vi "CRYGet Phase Index.vi"(10 "SelectedRow":i32[](array[numeric]), 11 "Legend Ref":refnum<vi>) -> (2 "CurveLibIndex":i32[](array[numeric]), 3 "LegendIndex":i32[](array[numeric]))   [LabVIEW 2013]
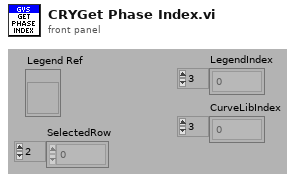
[diagram p1: front panel]
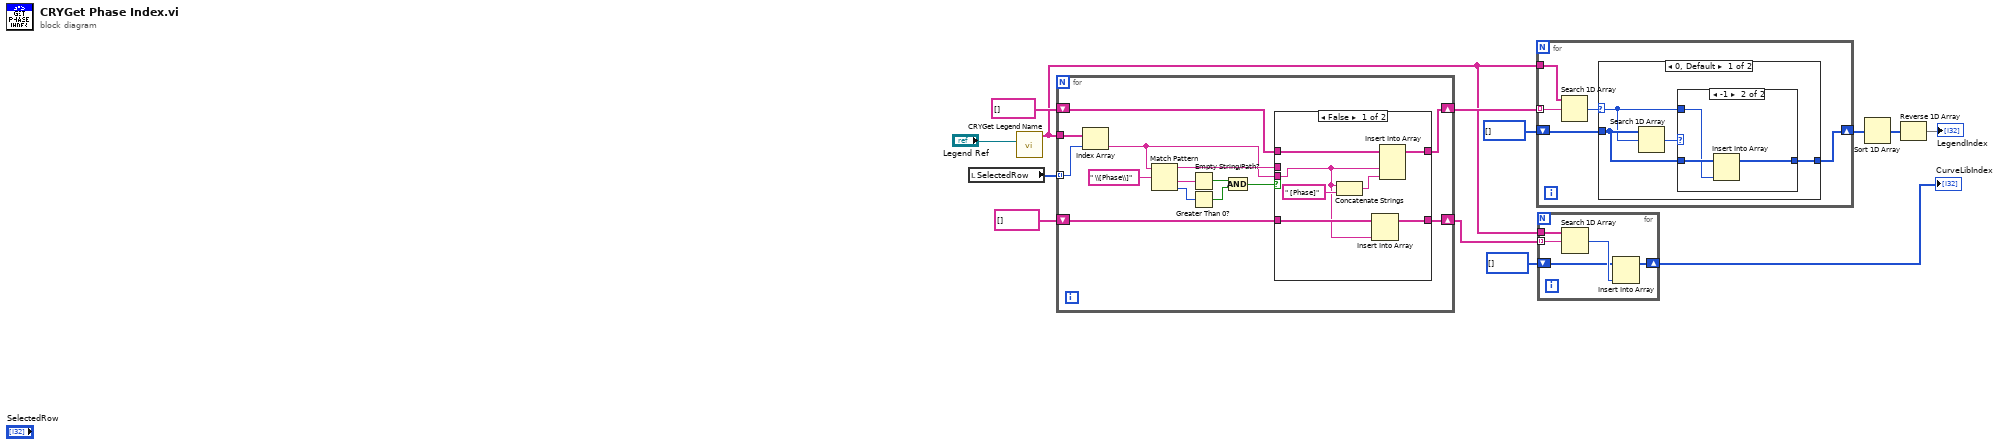
[diagram p0: block diagram]
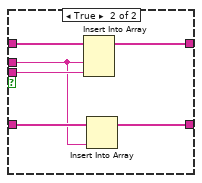
[diagram p4: hidden frame]
diagram:
  n1 = local read "SelectedRow"() -> (w13:i32[])
  n2 = call "CRYGet Legend Name.vi"("MCListbox Refnum"="Legend Ref") -> ("Names Out"=w3:string[])  [unwired: 10 in]
  n3 = for {
    tunnel: w13 -> [w26] mode=indexing
    tunnel: w3 -> [w27]
    shift-right: [w16] -> w11
    shift-left: string[] [] ("Names Out") -> [w18]
    shift-right: [w14] -> w2
    shift-left: string[] [] ("Names Out") -> [w15]
    n4 = Index Array(array=w27, index=w26) -> (element=w17:string)
    n5 = Match Pattern(string=w17, regular expression=" \\[Phase\\]") -> (before substring=w19:string, after substring=w22:string, offset past match=w23:i32)  [unwired: 1 in, 1 out]
    n6 = Empty String/Path?(string/path=w22) -> (empty?=w24:bool)
    n7 = Greater Than 0?(x=w23) -> (x > 0?=w25:bool)
    n8 = And(x=w24, y=w25) -> (x .and. y?=w20:bool)
    n9 = case shown="False" w20 {
      tunnel: w19 -> [_ w35]
      tunnel: w18 -> [w34 w40]
      tunnel: w17 -> [w28 w39]
      tunnel: [w31 w38] -> w16
      tunnel: w15 -> [w30 w37]
      tunnel: [w29 w36] -> w14
      frame False {
        n10 = Concatenate Strings(w28, " [Phase]" ("regular expression")) -> (w32:string)
        n11 = Insert Into Array(array=w30, new element=w28) -> (w29:string[])  [unwired: 1 in]
        n12 = Insert Into Array(array=w34, new element #1=w28, new element #2=w32) -> (w31:string[])  [unwired: 1 in]
      }
      frame True {
        n13 = Insert Into Array(array=w40, new element #1=w35, new element #2=w39) -> (w38:string[])  [unwired: 1 in]
        n14 = Insert Into Array(array=w37, new element=w35) -> (w36:string[])  [unwired: 1 in]
      }
    }
  }
  n15 = for {
    tunnel: w3 -> [w45]
    tunnel: w11 -> [w44] mode=indexing
    shift-right: [w41] -> w8
    shift-left: i32[] [] ("SelectedRow") -> [w42]
    n16 = Search 1D Array(1D array=w45, element=w44) -> (index of element=w43:i32)  [unwired: 1 in]
    n17 = case shown="0, Default" w43 {
      selector: w43 -> [w47 _]
      tunnel: w42 -> [w48 w54]
      tunnel: [w46 w54] -> w41
      frame 0, Default {
        n18 = Search 1D Array(1D array=w48, element=w47) -> (index of element=w49:i32)  [unwired: 1 in]
        n19 = case shown="-1" w49 {
          tunnel: w48 -> [w50 w53]
          tunnel: w47 -> [_ w52]
          tunnel: [w50 w51] -> w46
          frame 0, Default {
          }
          frame -1 {
            n20 = Insert Into Array(array=w53, new element=w52) -> (w51:i32[])  [unwired: 1 in]
          }
        }
      }
      frame -1 {
      }
    }
  }
  n21 = for {
    tunnel: w3 -> [w59]
    tunnel: w2 -> [w58] mode=indexing
    shift-right: [w55] -> w1
    shift-left: i32[] [] ("SelectedRow") -> [w56]
    n22 = Search 1D Array(1D array=w59, element=w58) -> (index of element=w57:i32)  [unwired: 1 in]
    n23 = Insert Into Array(array=w56, new element=w57) -> (w55:i32[])  [unwired: 1 in]
  }
  "CurveLibIndex" <- w1
  n24 = Sort 1D Array(array=w8) -> (sorted array=w7:i32[])
  n25 = Reverse 1D Array(array=w7) -> (reversed array=→"LegendIndex":i32[])
